vi "Write SamplesPerRep.vi"(8 "error in (no error)":errorcluster, 10 "SamplesPerRep":u16=4000, 11 "tCRD in":refnum<class "Open Path CRD.lvclass">) -> (0 "error out":errorcluster, 3 "tCRD out":refnum<class "Open Path CRD.lvclass">)   [LabVIEW 2015, in "Open Path CRD.lvclass"]
uses:
  Open Path CRD.lvclass
  Open Path CRD.lvclass/Open Path CRD.ctl
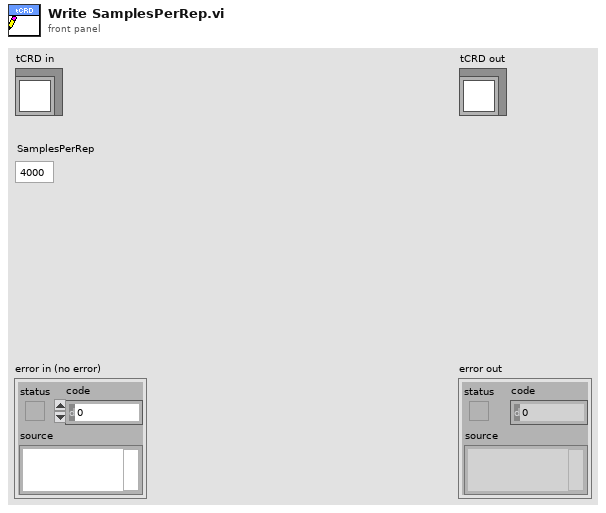
[diagram p1: front panel]
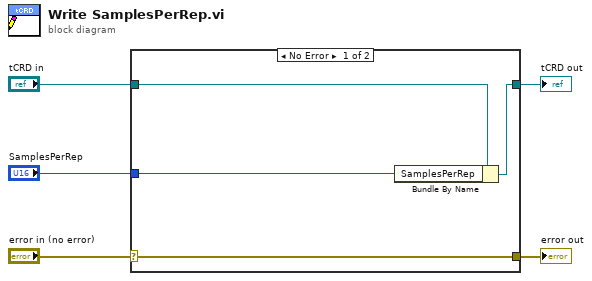
[diagram p0: block diagram]
diagram:
  n1 = case shown="No Error" "error in (no error)" {
    selector: "error in (no error)" -> [w9 w10]
    tunnel: [w9 w10] -> w4
    tunnel: [w7 w11] -> w2
    tunnel: "tCRD in" -> [w8 w11]
    tunnel: "SamplesPerRep" -> [w6 _]
    frame No Error {
      n2 = Bundle By Name(cluster=w8, "SamplesPerRep"=w6) -> (w7:refnum<class "Open Path CRD.lvclass">)
    }
    frame Error {
    }
  }
  "error out" <- w4
  "tCRD out" <- w2
